vi "Dkm To Skm.vi"(8 "error in (no error)":errorcluster, 11 "dKilo":dbl) -> (0 "error out":errorcluster, 3 "dkm_STR":string)   [LabVIEW 2023, in "POSCONV.lvlib"]
doc: "Converts double kilometres to double kilometres STRING...\n\n\nchar *DkmToSkm(double dKilo);"
uses:
  POSCONV.lvlib
  C:/Users/J Gordon/Documents/Rail Tech/TV-HR/02 - Code/Modules/POSCONV/POSCONV.dll
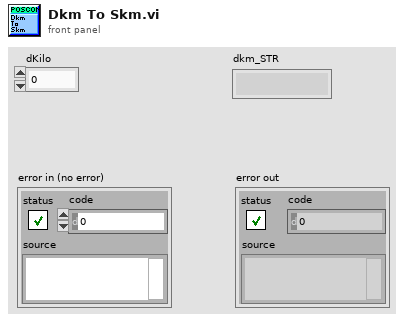
[diagram p1: front panel]
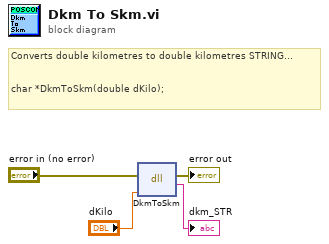
[diagram p0: block diagram]
diagram:
  # "Converts double kilometres to double kilometres STRING...\n\n\nchar *DkmToSkm(double dKilo);"
  n1 = dll-call lib="C:/Users/J Gordon/Documents/Rail Tech/TV-HR/02 - Code/Modules/POSCONV/POSCONV.*" fn="DkmToSkm"(error in="error in (no error)", "dKilo"="dKilo") -> (error out=→"error out":errorcluster, →"dkm_STR":string)  [unwired: 3 in, 1 out]
